vi "MGI Disable Enum Grayed Merge VI.vi"   [LabVIEW 2020]
doc: "The Disable Enum.vi is smaller than the Enum \"Disabled and Greyed out\" and may be dropped on block diagrams to conserve space."
uses:
  <userlib>/_MGI/Application Control/MGI Disable Enum/MGI Disable Enum (Grayed).vi
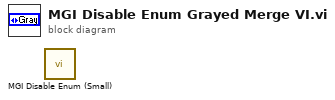
[diagram p0: block diagram]
diagram:
  n1 = call-poly <userlib>:"MGI Disable Enum (Small).vi"() -> ()  [unwired: 1 out]
